vi "NPC3SG Set Voltage v10.6.1.vi"(2 "Voltage":dbl format="%.2f", 3 "Axis":i32=1 min=0 max=2 step=1, 4 "Drive Visa Name":refnum<visa-resource-name>="COM5") -> (0 "Send Error":errorcluster caption="Fehler (Ausgang)")   [LabVIEW 2010]
uses:
  drivers/Newport NPC3SG/SubNPC3SG.llb/device variables.vi
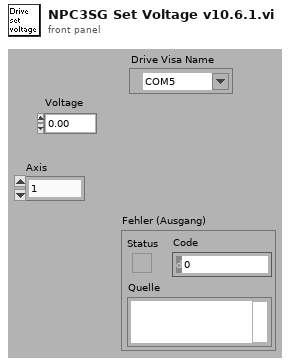
[diagram p1: front panel]
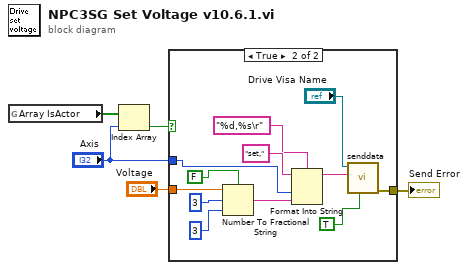
[diagram p0: block diagram]
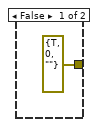
[diagram p2: hidden frame]
diagram:
  n1 = global read "device variables.vi" "Array IsActor"() -> (w5:bool[])
  n2 = Index Array(array=w5, index="Axis") -> (element=w4:bool)
  n3 = case shown="True" w4 {
    tunnel: "Axis" -> [_ w11]
    tunnel: [errorcluster {"status"=TRUE, "code"=0, "source"=""} ("error out") w10] -> w3
    tunnel: "Voltage" -> [_ w8]
    frame False {
    }
    frame True {
      n4 = Number To Fractional String(use system decimal point (T)=FALSE ("Systemdezimalzeichen verwenden (T)"), number=w8, width (-)=i16 3 ("Breite (-)"), precision (6)=i16 3 ("Genauigkeit (6)")) -> (F-format string=w17:string)
      n5 = Format Into String(format string="%d,%s\r", initial string="set,", w11, w17) -> (resulting string=w18:string)  [unwired: 1 in, 1 out]
      n6 = call "senddata.vi"("read ERR"=TRUE, "writebuffer"=w18, "VISA-Ressourcen-Name"="Drive Visa Name") -> ("error out"=w10:errorcluster)  [unwired: 6 in, 2 out]
    }
  }
  "Send Error" <- w3
